vi "GetJSONData.vi"(0 "reference in":refnum<class "Object.lvclass">, 2 "VI Reference":refnum<vi>, 5 "error in (no error)":errorcluster) -> (14 "reference out":refnum<class "Object.lvclass">, 15 "JSON string":string, 19 "error out":errorcluster)   [LabVIEW 2014, in "Object.lvclass"]
uses:
  Object.lvclass
panel:
  in  "numnum":dbl format="%.15g"
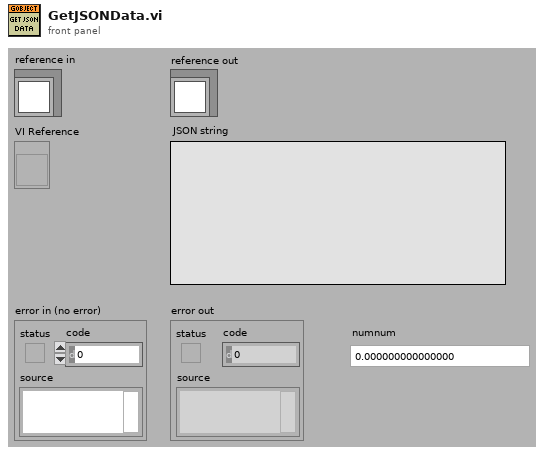
[diagram p1: front panel]
types:
  T1 = typedef "Object.lvclass/Attributes.ctl" = cluster{"UID":i32, "Type":string, "Coordinates":T2}
  T2 = typedef "Object.lvclass/Coordinates.ctl" = cluster{"Left":i32, "Top":i32, "Height":u32, "Width":u32}
  T3 = typedef "Type Descriptor Enumeration__ogtk.ctl" = enum8{"<Null>", "I8", "I16", "I32", "I64", "U8", "U16", "U32", "U64", "SGL", "DBL", "EXT", "CSG", "CDB", "CXT", "0x0F", "0x10", "0x11", "0x12", "0x13", "0x14", "Enum U8", "Enum U16", "Enum U32", "Enum U64", "SGL PQ", "DBL PQ", "EXT PQ", "CSG PQ", "CDB PQ", "CXT PQ", "0x1F", "0x20", "Boolean", "0x22", "0x23", "0x24", "0x25", "0x26", "0x27", "0x28", "0x29", "0x2A", "0x2B", "0x2C", "0x2D", "0x2E", "0x2F", "String", "0x31", "Path", "Pict", "0x34", "0x35", "0x36", "DAQ", "0x38", "0x39", "0x3A", "0x3B", "0x3C", "0x3D", "0x3E", "0x3F", "Array", "0x41", "0x42", "0x43", "0x44", "0x45", "0x46", "0x47", "0x48", "0x49", "0x4A", "0x4B", "0x4C", "0x4D", "0x4E", "0x4F", "Cluster", "0x51", "0x52", "Variant", "Waveform", "0x55", "0x56", "0x57", "0x58", "0x59", "0x5A", "0x5B", "0x5C", "0x5D", "0x5E", "0x5F", "0x60", "0x61", "0x62", "0x63", "0x64", "0x65", "0x66", "0x67", "0x68", "0x69", "0x6A", "0x6B", "0x6C", "0x6D", "0x6E", "0x6F", "Refnum"}
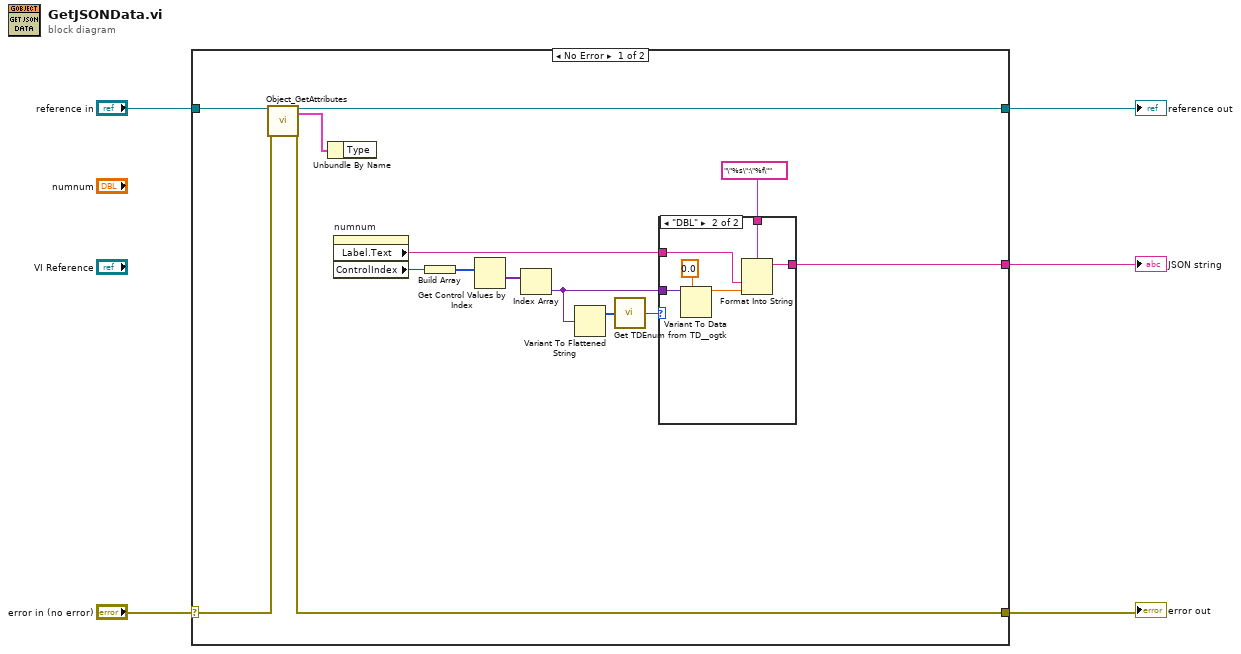
[diagram p0: block diagram]
diagram:
  n1 = case shown="No Error" "error in (no error)" {
    selector: "error in (no error)" -> [w19 w27]
    tunnel: [w17 w27] -> w4
    tunnel: [w15 w26] -> w2
    tunnel: "reference in" -> [w16 w26]
    tunnel: [w6 _] -> w1
    frame No Error {
      n2 = call "Object_GetAttributes.vi"("reference in"=w16, "error in (no error)"=w19) -> ("reference out"=w15:refnum<class "Object.lvclass">, "Data"=w18:T1, "error out"=w17:errorcluster)  [unwired: 14 in, 1 out]
      n3 = Unbundle By Name(w18) -> ()  [unwired: 1 out]
      n4 = property on="numnum" class="DigNum (strict)"() -> ("Label.Text"=w7:string, "ControlIndex"=w14:i32)  [unwired: 2 in, 2 out]
      n5 = Build Array(w14) -> (w13:i32[])
      n6 = Get Control Values by Index(1:w13) -> (10:w12:variant[])  [unwired: 2 in, 1 out]
      n7 = Index Array(array=w12) -> (element=w9:variant)  [unwired: 1 in]
      n8 = Variant To Flattened String(Variant=w9) -> (1:w11:i16[])  [unwired: 1 out]
      n9 = call <userlib>:"Get TDEnum from TD__ogtk.vi"("Type Descriptor"=w11) -> ("Type Descriptor Enumeration"=w10:T3)  [unwired: 4 in]
      n10 = case shown="\"DBL\"" w10 {
        tunnel: w9 -> [_ w25]
        tunnel: "\"%s\":\"%f\"" -> [_ w23]
        tunnel: w7 -> [_ w22]
        tunnel: [_ w20] -> w6
        frame "<Null>", Default {
        }
        frame "DBL" {
          n11 = Variant To Data(type=0.0, Variant=w25) -> (data=w21:dbl)  [unwired: 1 in, 1 out]
          n12 = Format Into String(format string=w23, w22, w21) -> (resulting string=w20:string)  [unwired: 2 in, 1 out]
        }
      }
    }
    frame Error {
    }
  }
  "error out" <- w4
  "reference out" <- w2
  "JSON string" <- w1
